vi "query_cmd.vi"(8 "error in (no error)":errorcluster, 10 "write buffer":string, 11 "VISA Refnum in":refnum<visa-resource-name>) -> (0 "error out":errorcluster, 2 "String":string, 3 "VISA Refnum out":refnum<visa-resource-name>)   [LabVIEW 2018]
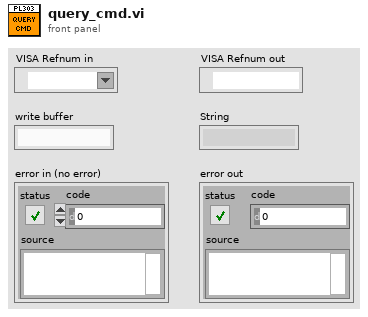
[diagram p1: front panel]
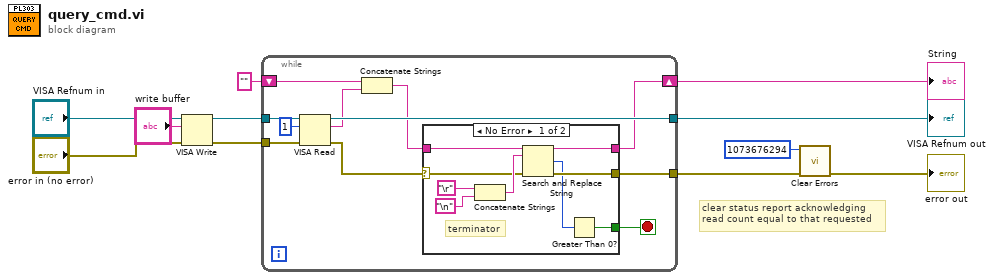
[diagram p0: block diagram]
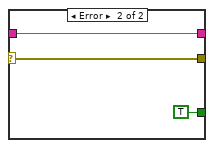
[diagram p2: hidden frame]
diagram:
  # "clear status report acknowledging\nread count equal to that requested"
  n1 = VISA Write(VISA resource name="VISA Refnum in", write buffer="write buffer", error in (no error)="error in (no error)") -> (VISA resource name out=w6:refnum<visa-resource-name>, error out=w5:errorcluster)  [unwired: 1 out]
  n2 = while {
    tunnel: w6 -> [w19]
    tunnel: [w22] -> w1
    tunnel: w5 -> [w20]
    tunnel: [w16] -> w9
    shift-right: [w12] -> w8
    shift-left: "" -> [w17]
    stop <- w14 stop-if-true
    n3 = VISA Read(VISA resource name=w19, byte count=u32 1, error in (no error)=w20) -> (VISA resource name out=w22:refnum<visa-resource-name>, read buffer=w18:string, error out=w15:errorcluster)  [unwired: 1 out]
    n4 = Concatenate Strings(w17, w18) -> (w13:string)
    n5 = case shown="No Error" w15 {
      selector: w15 -> [w25 w34]
      tunnel: [w31 w34] -> w16
      tunnel: w13 -> [w30 w32]
      tunnel: [w24 TRUE] -> w14
      tunnel: [w23 w32] -> w12
      frame No Error {
        # "terminator"
        n6 = Concatenate Strings("\r", "\n") -> (w27:string)
        n7 = Search and Replace String(input string=w30, search string=w27, error in=w25) -> (result string=w23:string, number of replacements=w26:i32, error out=w31:errorcluster)  [unwired: 5 in, 1 out]
        n8 = Greater Than 0?(x=w26) -> (x > 0?=w24:bool)
      }
      frame Error {
      }
    }
  }
  "String" <- w8
  "VISA Refnum out" <- w1
  n9 = call <vilib>:"Clear Errors.vi"("error in (no error)"=w9, "specific error code to clear (0: all)"=1073676294) -> ("error out"=→"error out":errorcluster)  [unwired: 4 in, 1 out]
